vi "Run.vi"(8 "error in (no error)":errorcluster caption="entrée d'erreur (pas d'erreur)", 11 "ParameterSampler.lvclass":refnum<class "ParameterSampler.lvclass">) -> (0 "error out":errorcluster caption="sortie d'erreur", 2 "Data":string[][](array[string]), 3 "ParameterSampler.lvclass":refnum<class "ParameterSampler.lvclass">)   [LabVIEW 2020, in "ParameterSampler.lvclass"]
doc: "Returns :\n\n- params : dict of str to any\n Yields dictionaries mapping each estimator parameter to as sampled value."
uses:
  ParameterSampler.lvclass
  ParameterSampler.lvclass/ParameterSampler.ctl
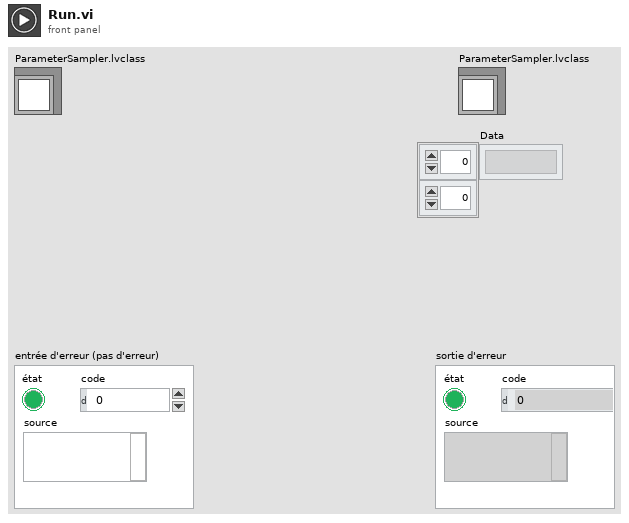
[diagram p1: front panel]
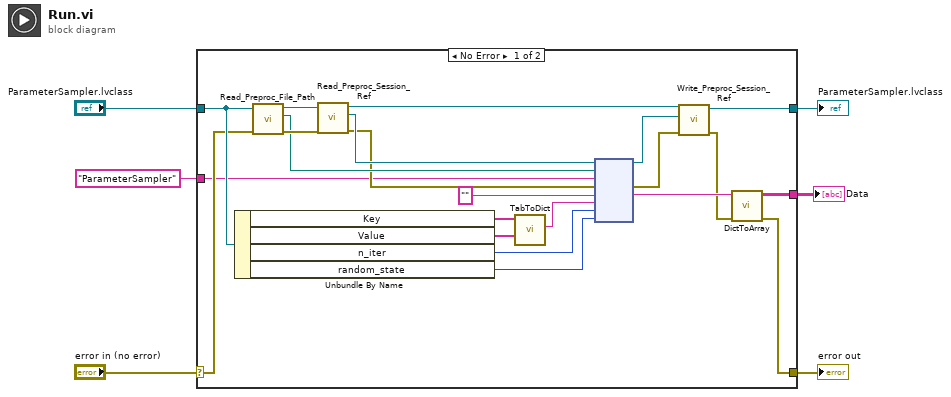
[diagram p0: block diagram]
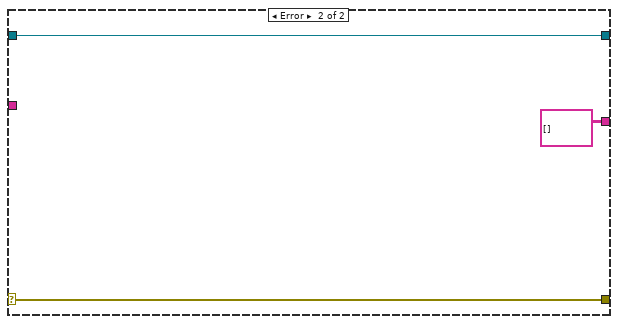
[diagram p2: hidden frame]
diagram:
  n1 = case shown="No Error" "error in (no error)" {
    selector: "error in (no error)" -> [w18 w31]
    tunnel: [w7 w31] -> w5
    tunnel: [w14 w30] -> w3
    tunnel: "ParameterSampler.lvclass" -> [w19 w30]
    tunnel: "ParameterSampler" -> [w17 _]
    tunnel: [w9 string[][] [] ("String 2DArray")] -> w1
    frame No Error {
      n2 = Unbundle By Name(w19) -> ("Key"=w13:string[], "Value"=w12:string[], "n_iter"=w16:i32, "random_state"=w15:i32)
      n3 = call-dynamic "Read_Preproc_File_Path.vi"("error in (no error)"=w18, "Python in"=w19) -> ("error out"=w27:errorcluster, "File_Path"=w26:path, "Python out"=w28:refnum<class "ParameterSampler.lvclass">)  [unwired: 7 in]
      n4 = call-dynamic "Read_Preproc_Session_Ref.vi"("error in (no error)"=w27, "Python in"=w28) -> ("error out"=w24:errorcluster, "Session_ref"=w25:refnum<k35>, "Python out"=w23:refnum<class "ParameterSampler.lvclass">)  [unwired: 7 in]
      n5 = call "TabToDict.vi"("String Value"=w12, "String key"=w13) -> ("Dict with string value"=w11:string)  [unwired: 8 in, 1 out]
      n6 = node(w25, w26, w17, w24, "", w11, w16, w15) -> (w21:refnum<k35>, w22:errorcluster, w10:string)  [unwired: 3 in, 2 out]
      n7 = call-dynamic "Write_Preproc_Session_Ref.vi"("error in (no error)"=w22, "Session_ref"=w21, "Python in"=w23) -> ("error out"=w8:errorcluster, "Python out"=w14:refnum<class "ParameterSampler.lvclass">)  [unwired: 7 in]
      n8 = call "DictToArray.vi"("entrée d'erreur (pas d'erreur)"=w8, "Dict"=w10) -> ("sortie d'erreur"=w7:errorcluster, "String 2DArray"=w9:string[][])  [unwired: 8 in]
    }
    frame Error {
    }
  }
  "error out" <- w5
  "ParameterSampler.lvclass" <- w3
  "Data" <- w1
